vi "FTW-Container-Support-XML-PopulateNode.vi"(0 "Element Node":refnum<k20>, 5 "JSON":string, 11 "error in":errorcluster) -> (4 "Element Node out":refnum<k20>, 6 "Serialized Node":string, 15 "error out":errorcluster)   [LabVIEW 2012, in "FTW-Container.lvclass"]
uses:
  FTW-Container.lvclass
  JSON/FTW-JSON-CompositeType.ctl
  JSON/FTW-JSON-RegexParse.vi
  Regex/FTW-Regex.vi
  JSON/FTW-JSON-RegexHeader.vi
  Error/FTW-ERR-ThrowError.vi
  Error/FTW-ERR-StatusError.vi
  JSON/FTW-JSON-Unescape.vi
  <resource>/objmgr/DOMUserDefRef.rc
panel:
  # "Inputs"
  # "Outputs"
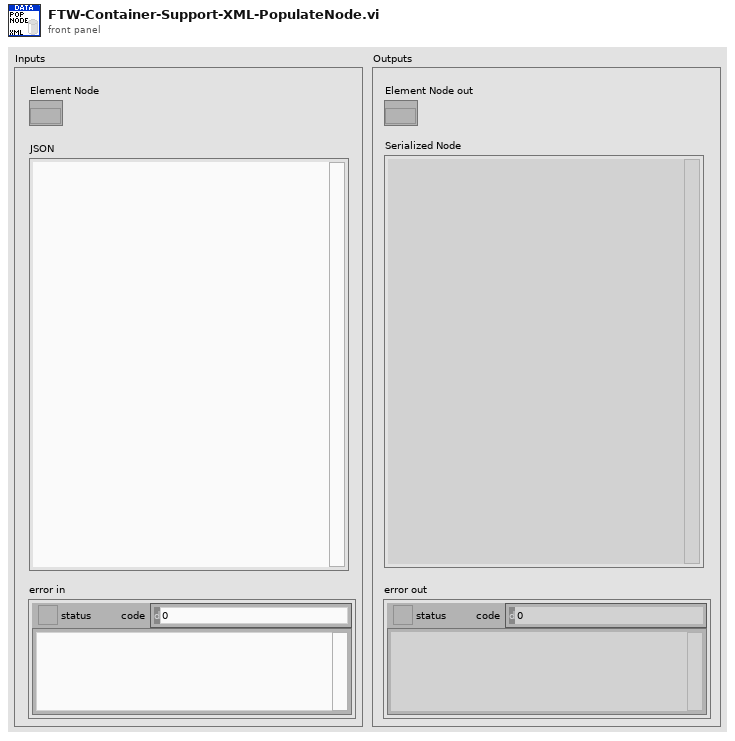
[diagram p1: front panel]
types:
  T1 = typedef "FTW-JSON-CompositeType.ctl" = enum16{"Object", "Array"}
  T2 = typedef "FTW-Container.lvclass/FTW-Container-Support-JSON-ElementToProcess.ctl" = cluster{"Name":string, "Value":string, "JSON Type":T3}
  T3 = typedef "FTW-JSON-Datatype.ctl" = enum16{"Object", "Array", "String", "Number", "Boolean", "NULL", "<Refnum>", "<Enum>", "<Unknown>"}
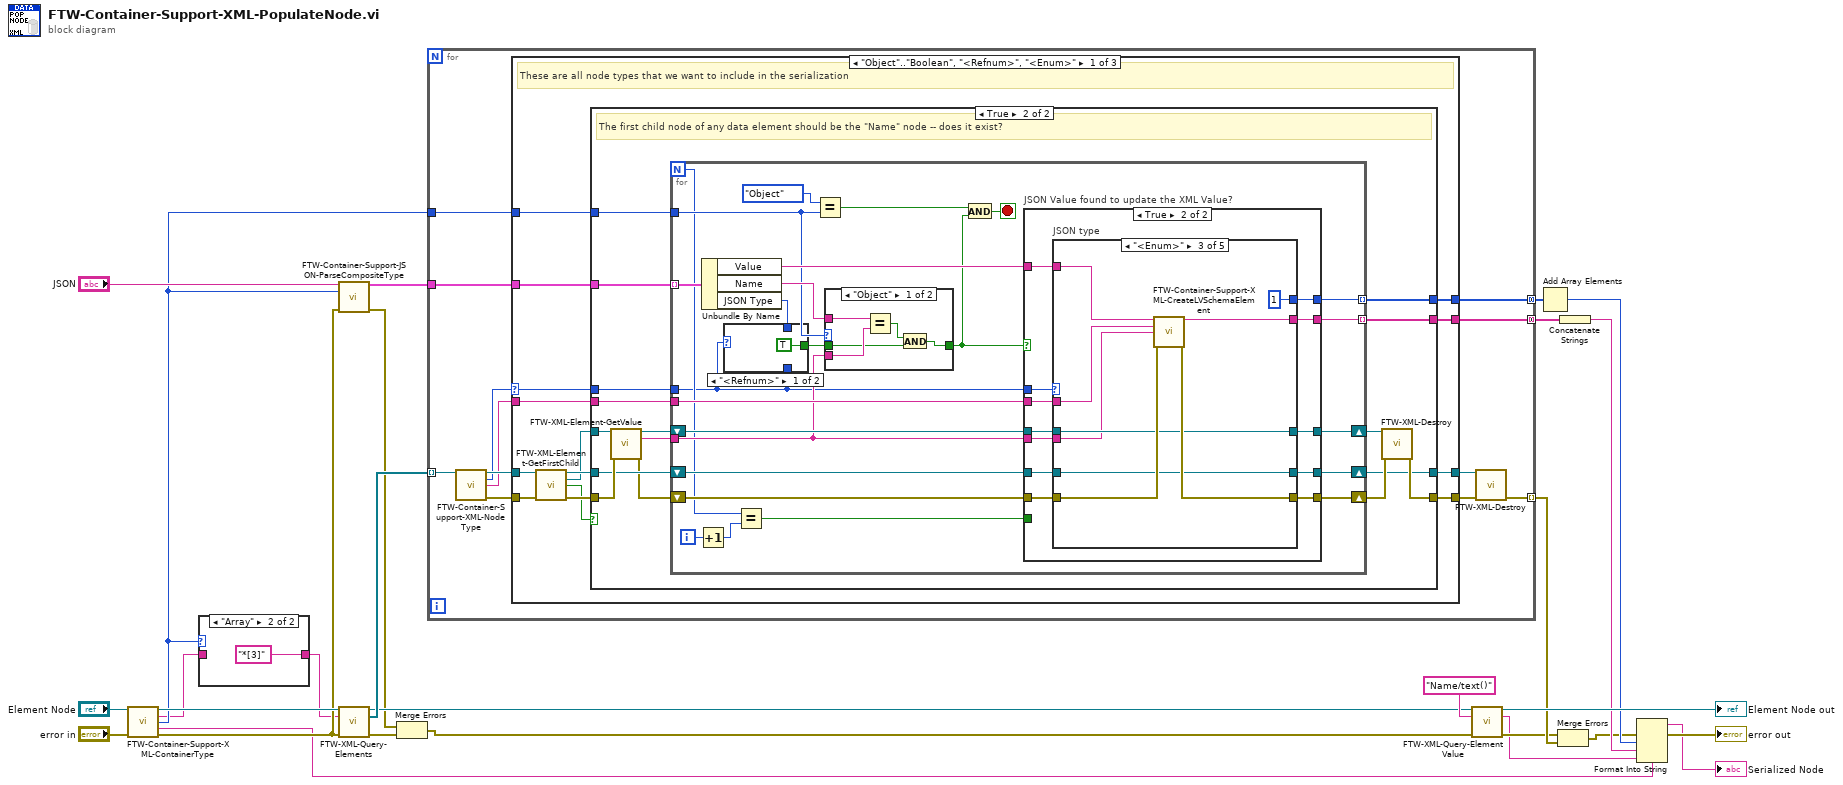
[diagram p0: block diagram]
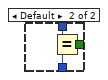
[diagram p4: hidden frame]
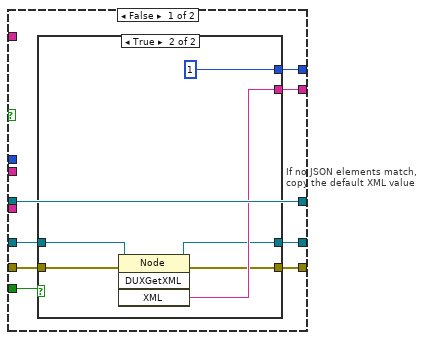
[diagram p6: hidden frame]
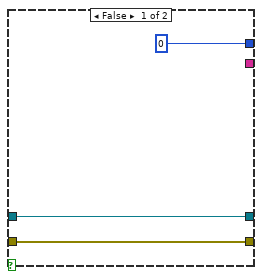
[diagram p7: hidden frame]
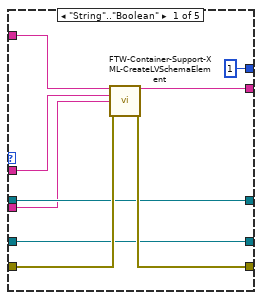
[diagram p8: hidden frame]
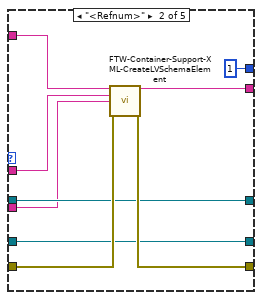
[diagram p9: hidden frame]
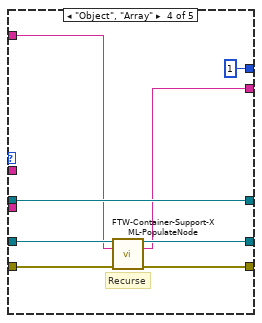
[diagram p10: hidden frame]
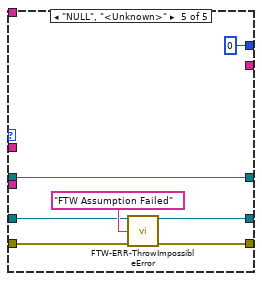
[diagram p11: hidden frame]
diagram:
  n1 = call "FTW-Container-Support-XML-ContainerType.vi"("Element Node"="Element Node", "error in"="error in") -> ("Element Node out"=w8:refnum<k20>, "Parent XPath Query"=w2:string, "Parent Type"=w3:T1, "XML Structure"=w4:string, "error out"=w5:errorcluster)  [unwired: 9 in]
  n2 = case shown="\"Array\"" w3 {
    tunnel: w2 -> [w28 _]
    tunnel: [w28 "*[3]"] -> w1
    frame Default {
    }
    frame "Array" {
    }
  }
  n3 = call "FTW-Container-Support-JSON-ParseCompositeType.vi"("JSON String"="JSON", "Expected Type"=w3, "error in"=w5) -> ("Elements"=w23:T2[], "error out"=w11:errorcluster)  [unwired: 11 in]
  n4 = call "FTW-XML-Query-Elements.vi"("XML Node"=w8, "XPath Query"=w1, "error in"=w5) -> ("XML Node out"=w17:refnum<k20>, "Matching Nodes"=w19:refnum<k20>[], "error out"=w10:errorcluster)  [unwired: 9 in, 1 out]
  n5 = Merge Errors(w11, w10) -> (w9:errorcluster)
  n6 = for {
    tunnel: w19 -> [w41] mode=indexing
    tunnel: [w38] -> w20 mode=concatenating
    tunnel: [w37] -> w18 mode=indexing
    tunnel: w23 -> [w32]
    tunnel: [w31] -> w21 mode=concatenating
    tunnel: w3 -> [w30]
    n7 = call "FTW-Container-Support-XML-NodeType.vi"("Element Node"=w41) -> ("Element Node out"=w40:refnum<k20>, "JSON Type"=w35:T3, "Node XML Type"=w33:string, "error out"=w39:errorcluster)  [unwired: 11 in]
    n8 = case shown="\"Object\"..\"Boolean\", \"<Refnum>\", \"<Enum>\"" w35 {
      selector: w35 -> [w49 _ _]
      tunnel: w39 -> [w47 w179 w182]
      tunnel: [w50 w179 w182] -> w36
      tunnel: w40 -> [w48 w180 w181]
      tunnel: [w51 _ _] -> w38
      tunnel: [w52 w180 w181] -> w34
      tunnel: w33 -> [w45 _ _]
      tunnel: w32 -> [w46 _ _]
      tunnel: [w44 _ _] -> w31
      tunnel: w30 -> [w43 _ _]
      frame "Object".."Boolean", "<Refnum>", "<Enum>" {
        # "These are all node types that we want to include in the serialization"
        n9 = call "FTW-XML-Element-GetFirstChild.vi"("Element Node"=w48, "error in"=w47) -> ("Element Node out"=w53:refnum<k20>, "First Child Element Node"=w42:refnum<k20>, "Found?"=w54:bool, "error out"=w55:errorcluster)  [unwired: 10 in]
        n10 = case shown="True" w54 {
          tunnel: w53 -> [w56 w66]
          tunnel: w55 -> [w57 w72]
          tunnel: w49 -> [_ w63]
          tunnel: [w56 w67] -> w52
          tunnel: [w57 w71] -> w50
          tunnel: [_ w69] -> w51
          tunnel: w46 -> [_ w70]
          tunnel: w45 -> [_ w62]
          tunnel: [_ w60] -> w44
          tunnel: w43 -> [_ w59]
          tunnel: w42 -> [_ w58]
          frame False {
            # "A child node did not exist; therefore it does not need to be destroyed"
          }
          frame True {
            # "The first child node of any data element should be the \"Name\" node -- does it exist?"
            n11 = call "FTW-XML-Element-GetValue.vi"("XML Node"=w58, "error in"=w72) -> ("XML Node out"=w64:refnum<k20>, "Node Text Value"=w61:string, "error out"=w65:errorcluster)  [unwired: 11 in]
            n12 = for {
              N -> [w78]
              tunnel: w70 -> [w98] mode=indexing
              tunnel: [w97] -> w69 mode=indexing
              tunnel: w63 -> [w74]
              tunnel: w62 -> [w90]
              tunnel: w61 -> [w88]
              shift-right: [w96] -> w68
              shift-left: w64 -> [w91]
              shift-right: [w95] -> w67
              shift-left: w66 -> [w93]
              shift-right: [w94] -> w73
              shift-left: w65 -> [w92]
              tunnel: [w84] -> w60 mode=indexing
              tunnel: w59 -> [w83]
              i -> [w77]
              stop <- w79 stop-if-true
              n13 = Increment(x=w77) -> (x+1=w76:i32)
              n14 = Unbundle By Name(w98) -> ("Value"=w89:string, "Name"=w87:string, "JSON Type"=w86:T3)
              n15 = case shown="\"<Refnum>\"" w74 {
                tunnel: w74 -> [_ w102]
                tunnel: w86 -> [_ w101]
                tunnel: [TRUE w100] -> w85
                frame "<Refnum>" {
                }
                frame Default {
                  n16 = Equal?(x=w101, y=w102) -> (x = y?=w100:bool)
                }
              }
              n17 = Equal?(x=w78, y=w76) -> (x = y?=w75:bool)
              n18 = Equal?(x=FTW-JSON-CompositeType."Object", y=w83) -> (x = y?=w81:bool)
              n19 = case shown="\"Object\"" w83 {
                tunnel: w88 -> [w107 _]
                tunnel: [w106 w108] -> w80
                tunnel: w87 -> [w105 _]
                tunnel: w85 -> [w103 w108]
                frame "Object" {
                  n20 = Equal?(x=w105, y=w107) -> (x = y?=w104:bool)
                  n21 = And(x=w104, y=w103) -> (x .and. y?=w106:bool)
                }
                frame "Array" {
                }
              }
              n22 = And(x=w81, y=w80) -> (x .and. y?=w79:bool)
              n23 = case "JSON Value found to update the XML Value?" shown="True" w80 {
                tunnel: [w116 w137] -> w97
                tunnel: [w115 w136] -> w96
                tunnel: [w113 w135] -> w95
                tunnel: [w111 w134] -> w94
                tunnel: w93 -> [w114 w133]
                tunnel: w92 -> [w112 w132]
                tunnel: w91 -> [w115 w131]
                tunnel: w74 -> [_ w130]
                tunnel: w90 -> [_ w129]
                tunnel: w89 -> [_ w128]
                tunnel: w88 -> [_ w127]
                tunnel: [w110 w126] -> w84
                tunnel: w75 -> [w109 _]
                frame False {
                  n24 = case "If no JSON elements match,\ncopy the default XML value" shown="True" w109 {
                    tunnel: [_ w125] -> w116
                    tunnel: w114 -> [w119 w124]
                    tunnel: [w119 w123] -> w113
                    tunnel: w112 -> [w118 w122]
                    tunnel: [w118 w121] -> w111
                    tunnel: [0 1] -> w110
                    frame False {
                    }
                    frame True {
                      n25 = invoke class="Node" method="DUXGetXML"(reference=w124, error in=w122) -> (reference out=w123:refnum<k20>, error out=w121:errorcluster, "XML"=w125:string)  [unwired: 2 in, 1 out]
                    }
                  }
                }
                frame True {
                  n26 = case "JSON type" shown="\"<Enum>\"" w130 {
                    tunnel: [w144 w153 w162 w169 w178] -> w134
                    tunnel: w133 -> [w141 w150 w159 w171 w174]
                    tunnel: [w141 w150 w159 w168 w174] -> w135
                    tunnel: w131 -> [w143 w152 w161 w172 w176]
                    tunnel: w132 -> [w145 w154 w163 w170 w175]
                    tunnel: [w143 w152 w161 w172 w176] -> w136
                    tunnel: [w146 w155 w164 w167 _] -> w137
                    tunnel: w127 -> [w139 w148 w157 _ _]
                    tunnel: w129 -> [w140 w149 w158 _ _]
                    tunnel: w128 -> [w142 w151 w160 w166 _]
                    tunnel: [1 1 1 1 0] -> w126
                    frame "String".."Boolean" {
                      n27 = call "FTW-Container-Support-XML-CreateLVSchemaElement.vi"("JSON Scalar Value"=w142, "Node LV Type"=w140, "Node Name"=w139, "error in"=w145) -> ("LV Schema Node"=w146:string, "error out"=w144:errorcluster)  [unwired: 10 in]
                    }
                    frame "<Refnum>" {
                      n28 = call "FTW-Container-Support-XML-CreateLVSchemaElement.vi"("JSON Scalar Value"=w151, "Node LV Type"=w149, "Node Name"=w148, "error in"=w154) -> ("LV Schema Node"=w155:string, "error out"=w153:errorcluster)  [unwired: 10 in]
                    }
                    frame "<Enum>" {
                      n29 = call "FTW-Container-Support-XML-CreateLVSchemaElement.vi"("JSON Scalar Value"=w160, "Node LV Type"=w158, "Node Name"=w157, "error in"=w163) -> ("LV Schema Node"=w164:string, "error out"=w162:errorcluster)  [unwired: 10 in]
                    }
                    frame "Object", "Array" {
                      # "Recurse"
                      n30 = call "FTW-Container-Support-XML-PopulateNode.vi"("Element Node"=w171, "JSON"=w166, "error in"=w170) -> ("Element Node out"=w168:refnum<k20>, "Serialized Node"=w167:string, "error out"=w169:errorcluster)  [unwired: 10 in]
                    }
                    frame "NULL", "<Unknown>" {
                      n31 = call "FTW-ERR-ThrowImpossibleError.vi"("Reason this error should never happen"="FTW Assumption Failed", "error in"=w175) -> ("error out"=w178:errorcluster)  [unwired: 13 in]
                    }
                  }
                }
              }
            }
            n32 = call "FTW-XML-Destroy.vi"("XML Node"=w68, "error in"=w73) -> ("error out"=w71:errorcluster)  [unwired: 13 in]
          }
        }
      }
      frame "NULL" {
        # "There is no mapping from LV to the JSON null type, therefore, we never expect this case."
      }
      frame "<Unknown>" {
        # "This case is most likely a node type in the LabVIEW Schema that is unnecessary to parse."
      }
    }
    n33 = call "FTW-XML-Destroy.vi"("XML Node"=w34, "error in"=w36) -> ("error out"=w37:errorcluster)  [unwired: 13 in]
  }
  n34 = call "FTW-XML-Query-ElementValue.vi"("XML Node"=w17, "XPath"="Name/text()", "error in"=w9) -> ("XML Node out"=→"Element Node out":refnum<k20>, "Value"=w15:string, "error out"=w16:errorcluster)  [unwired: 9 in, 1 out]
  n35 = Add Array Elements(numeric array=w21) -> (sum=w14:i32)
  n36 = Merge Errors(w16, w18) -> (w12:errorcluster)
  n37 = Concatenate Strings(w20) -> (w13:string)
  n38 = Format Into String(format string=w4, error in=w12, w14, w13, w15) -> (resulting string=→"Serialized Node":string, error out=→"error out":errorcluster)  [unwired: 1 in]
